vi "Day 10-1.vi"() -> ()   [LabVIEW 2020]
uses:
  Open Symbol.ctl
  <vilib>/regexp/Match Regular Expression.xnode
panel:
  out "Answer":u64
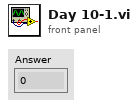
[diagram p1: front panel]
types:
  T1 = typedef "Open Symbol.ctl" = enum16{"(", "[", "{", "<"}
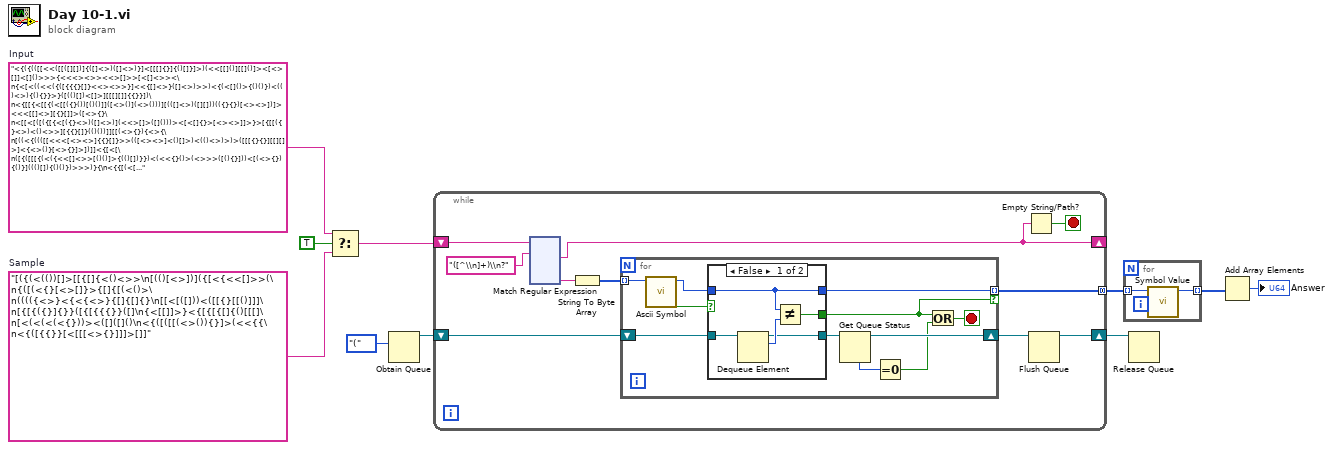
[diagram p0: block diagram]
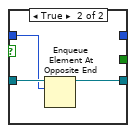
[diagram p2: hidden frame]
diagram:
  w9 = "[({(<(())[]>[[{[]{<()<>>\n[(()[<>])]({[<{<<[]>>(\n{([(<{}[<>[]}>{[]{[(<()>\n(((({<>}<{<{<>}{[]{[]{}\n[[<[([]))<([[{}[[()]]]\n[{[{({}]{}}([{[{{{}}([]\n{<[[]]>}<{[{[{[]{()[[[]\n[<(<(<(<{}))><([]([]()\n<{([([[(<>()){}]>(<<{{\n<{([{{}}[<[[[<>{}]]]>[]]"  # Sample
  w10 = "<{({(([[<<([[([][])]{([]<>)([]<>)}]<[[[]{}]{()[]}]>)(<<[[]()][[]()]><[<>[]]<[]()>>>{<<<><>><<>[]>>[<[]<>><\n{<[<((<<({([{{{}[]}<<><>>}]<<{[]<>}([]<>)>>)<{(<[]()>{()()})<(()<>){(){}}>}([(()[])<[]>][[[][]]{{}}])\n<{[[{<[[{(<[[({}())[()()]]([<>()](<>()))][(([]<>)([][]))(({}{})[<><>])]><<<[[]<>][{}[]]>([<>{}\n<[[<[([({[{<[({}<>)([]<>)](<<>[]>([]()))><[<[]{}>[<><>]]>}>[{[[({}<>)<()<>>][{{}[]}(()())]][[(<>{}){<>{\n[((<{((([[<<<[<><>]{{}[]}>>(([<><>]<()[]>)<(()<>)>)>([[[{}{}][[][]>]<{<>()}[<>{}]>])]]<{[<[\n([{([[[{(<({<<[]<>>[()()]>{(()[])}})<(<<{}()>(<>>>([(){}]))<[(<>{}){()}]((()[]){()()})>>>)}{\n<{{[(<[<<[[{<(()[])>[[{}()]{{}[]}]}[[(<>())[()()]]{<{}{}>}]](<{[<><>]{{}{}}}<({}[])[<><>]>><{[{}<>](<><>)\n{({<[<([[(({({<>()}{{}{}})})<<<((){})[[]()]><{{}()}[[][]]>>{(<{}{}>{{}()})}>)<<{<[{}[]][{}{}]>([[][]]{\n{[(((((<{[({<{()[]}(()())>{<(){}>{{}()}}}(<[<>()]{[]()}>(<()()>{{}<>})))[<[[{}{}](<>()>]({[]<>\n(([((<{<[((<{{<><>}{[]{}}}><<<<>>[{}]>([[]{}]<<>[]>)>)[[{<{}>{()()}}[[{}[]](()()>]](<<<>{}>[[]\n{<([[{<{([[<([[]<>]({}{})){{{}()}({}[])}>](<(<()()><()[]>)<<[]<>>([]{})>>)]){[{<<[()[]]<<>{}>><({\n<{[[([<<<(<{{(()<>)(()())}([{}<>]((){}))}>)>({({{{()<>}({}<>)}<[[]<>]{<>[]}>})(({<(){}>[<>[]]}<([]{})<[]{}>>)\n(<{<{[[({(<[((<>[]){{}})<(<><>)<[]{}>>]((<<>[]><[]()>)<<{}{}>{(){}}>)>(<[[[]<>]]{{<>{}}{[]()}}>(<{\n{(({{[[{<[((<<()<>>[{}{}]>((()<>){[]()})){{(<>{})[<>[]]}<<<><>>>}){{({<>{}}([]()))[{<><>}{[]\n(([<(([({{<{[{()<>}<{}[]>]}{[[()()][()<>]}[{<>{}}({}{})]}>((<<<>{}>[<>()]>{{[]<>}({}{})}){[<{\n[[{{(<<[[[[<<<<>{}>({}())>[([]<>)(()())]>]<<<{<>()}>[<<>[]>[()()]]>[([[]()]<[][]))<[<>{}]{{}<>\n{[{(((([<[{([(()()){()()}][<(){}>[{}<>)])[(<{}<>>{<>()})({{}<>}[()[]])]}(<({[]<>}<()[]>)({[]<>\n<<([(([{<{<<<[{}[]]((){})>((<>[])(()<>))>{{{<>()}{[]}}{([][])}}>[<{{<>[]}<<>>}({[]<>})>]]({({{<><>\n[{((<{<[[<[{[{{}<>}]{[{}][<>[]]}}[<([]())<()[]>>((<>){[]{}})]]<{(<()<>><{}<>]){[[]<>]({}{})}}({<{}[]>{{}\n<[<{(<[[<(((<({}[])><(<><>)(<>())]){{{()()}(<>())}<[{}()]>})[([[<>[]]{{}[]}]{{{}()}<{}[]>})[[(()<>){<>\n[([{{[<([{[([[()<>]])([[<>][()[]]][[<>[]]<<>[]>])]}{([<<{}()>({})>(<[]()>(<><>))]<<{{}<>}{<>}><(<>\n<<[[([([(<(<<[{}[]]<()[]]><{[]{}}[<>()]>>)>[<<({[][]}<<><>>)[<{}{}>{()<>}]><({<>{}}([]))((\n<({<{(<[({([[{()}(<><>)](<[][]>[{}{}])](([[]<>]<<>{}>))){({<<>{}>[[]{}]}<([][])>)<<(<><>)<[]<>>}>}}((([[()<\n{([<(<[(({[({[(){}]<<>{}>}[[{}{}][{}[]]])]{({[()<>]{()[]}}(<[][]>[()[]])){{{[]{}}(<>[])}[<(){}>(\n<[<[<{[{<[{[<<{}<>>(<>)>]{<({}{}){(){}}>((<>{})[{}<>])}}[<[[<><>]{{}<>}]{<()()>}>{<<[]()>(()())>{{{}<\n(({[[<<[({[{{<()()>}}{<[<>()]>}][(<{[][]}>{[{}()]{[]<>}})<{{<>{}}(()[])}{{[]()}<<>[]>}>]})\n<((<([[({(<{[[(){}]<[][]>]}>({<[()<>](()[])>(([]<>)([]<>))}<{[[]<>]{(){}}}(<()<>>([][]])>))}<{[<[({}\n{({{{[[{{[{(<<(){}>[{}{}]>((()<>)[<>{}]))[<<{}[]><[]>>[{{}{}}(<>[])]]}[(<<(){}>({}{}))((<>{})([]<>)))\n[[(({[{(<({[{<[]()>{()[]}}<(<>())<()()>>]<(({}[]){{}<>])((()<>){{}[]})>}([[({}{})[<>()]][{<><>}]]{([[\n[[{<[([<[((<([[]{}][{}<>])([{}<>])>[([()<>]{{}{}}){{[]()}}])<({{[]()}[[]()]))>)([<<<<>{}><{}()>><(<>\n<<({{{<{[<{<{<[]<>>[[]{}]}[<[]()>{[]{}}]>[[[(){}][<><>]]{(<>[]}({}{})}]}><[[({{}[]}{[]()}){(<>())[()<\n{{(({[[[{<[<(([]())([]{}))([{}{}](()[])}>]>}([<{[[[]()][(){}]]<{<>[]}>}({<()<>><[]<>>})>((([()\n(<(({{(([(({{<{}[]>({}())}([<>[]][{}()])}((<[][]>{()<>}){[[]<>]<{}{}>}))<({{[]<>}([][])}{<[]{}>{<>[]}})\n((([<([([{{{<<<>{}><{}[]>>[[<>[]][{}[]]]}}(([<<>{}>[()[]]][{{}{}}])(<[()()][<><>]>{{<>[]}})}}]<{[[<\n{{(<[<[<[<<[[(<>[])]({<><>}[()()])]>>]>[{{[[{(<>[])([][])}{[[][]]([]())}]>[[[<{}{}>({}())]<{<>\n<[{[[([[{[(<[<{}{}>{(){}}][{[]<>}<()[]]]>(([()<>][[][]]){[<>{}](()[])}))[[<<{}>[<>{}]>[({}{})({}{})]]<([[]{}\n({<<<{<({{{{{[()()]({}())}[[[]{}][<><>])}({<()()><[]()>}({<>()}))}{(((<>()){()()}){<(){}><()[]>})(([{}()]\n([<({[{({(<<{[{}()]}{{{}[]}((){})}>>)<<{[((){})[()]]}<<{[]<>}<<>()>>([<>()][[]<>])>>{<<[<>[]]<[]<>>)<{<\n(<[<<(<[[[[{{({}<>)[{}{}]}<[[]{}]([]<>)>}][<[<<>{}>{[]}][[[]{}](<>())]><<[<>()][(){}]><{[]\n(({[[(([<(([{({}[])[<>{}]}{(<>[])({}{})})<<<{}[]>({}())>[({}<>)<{}()>]>)[<<[[][]]((){})><{{}(\n{[((<([<[{[{<[<><>][()()]><{<>{}}>}[{<[][]>[()<>]}<(<>())<()<>>>]]<<<(<>())<()[]>>>[{{{}[]}}[[{}()]((){\n{{<{({{({[<((({}{}){<>[]}){<{}()>{<>[]}})>(<{<<>{}><[]<>>}>[[{[]<>>{<><>}]{((){})<(){}>}])]}(<{[{{<><>}{[\n(({<[[{[(<(((({}{}){()<>}))<{{[]{}}{{}{}}}<[{}<>][(){}]>>)>[{{(<<><>>([]{}))[((){})<{}[]>]}}(([[<>()]{<>()}]\n[<([[[<[<{<{<{[]{}}{[]{}}>[([]())<<>[]>]}({{[]{}}<[]()>}<({}())(<>{})>)>}[({[[{}[]][{}<>]]})]>]><[\n<{[<<[[<{[[{<<{}[]>[<><>]>}({[[]{}]<{}()>}((()[])))]{[<{()}[[]{}]>]{(({}[])<{}()>)<(<>())[()<>]\n[[([[{[[(([{[[<>()]{<>()}]({(){}}({}{}))}[<[<><>]([]())>(<[]()><{}[]>)]]{(<<<><>>[[]{}]>(<[][]>((){}))\n{(<<[[{[{{(<<<{}[]>(<>[])>({[]{}}([]{}))>[{<<>()>[[]<>]]([{}[]])])}[[{(<<><>>[()()])<<<><>>>}([<<>\n([((<(<[(<{((<{}{}>{<><>})){{(()[])[{}[]]}}}{[[[(){}][<><>]]]({<()<>>{{}[]}}<[()()]{()[]}>)}>[<{(<{}\n[(<[([[({({<[{<>()}([]<>)][(<><>)<()[]>]>})[{([(())({}[])][{[]<>}<()<>>])}({<[{}{}](()())><({}())[<>[]\n([(<<[<{<{((<(<>[])({}<>)>{{()()}<<>{}>}))<{[[()[]][()[]]][({}[])<{}()>]}{<({})><{[][]}{{}<>}>}>}<<<({(){}}\n[(<{(([({<{{(<[]<>>({}()))}}[<[[{}[]][[]]]>[({[]<>}(<>{}))]]>})]<([(<([[()()][[][]]]<((){}\n((({([(<<{{<<({}())(())>([<>()]<()()>)>}}<[(<{{}[]}<()<>>><({}{}){(){}}>)][(({()<>}([]()))([()]))({{{}()}\n{<(({[<([{[({([][])[[]{}]}<({}<>)<<>()>>)<<{<>()}{[]<>}>{{{}}{[]()}}>]}])<<{<(([[]{}]<<>[]>)){<<[]<>>><<()[\n[{<(<<<((<<<{[()<>]{[]<>}}>[[<{}{}>[()[]]]<(<><>)[()[]]>]>{[[[[]()][<>[]]]]({(<>}{[]{}}})}>){({\n<<[((<<[{{[(<[<>()]><{{}[]}{<>{}}>){[(()[])([]())][[(){}][{}[]]]}]([<[[][]]{(){}}><<{}{}>{<>{}}>][[\n{<<{<<{<({[[([<>{}])[{[]<>}{{}[]}]][[<()<>>[<>{}]]]]<([{[]()}({}{})]({[]()}{<>()})){[({}<>)[[]{}\n{<<[{((([<([[<[]()><<><>>][{()<>}<[][]>]]{<[{}[]][()[]]>[{<>{}>{[]}]}){[([[]{}]<()[]>)[[<>()][{}[]]\n({{{{<([[((({{{}{}}<()[]>}{<()<>>{{}<>}})(<({}{})>({<>{}}[[]()]))){(<<<><>><()[]>>[{()()}{[]<>}\n({<{[[{({{[<[{[][]}<[][]>]{(<><>)}>([[<>{}][<>{}]]({[]{}}<<>[]>))]}{[({[[]]{()[]}}{(<>{})[()()]})(<{(\n[{<<<[(<(<{((([]{}))[{<>()}[()[]]]){{<{}{}>}[<[]<>>{<>{}}]}}<(<[<>[]][()()]>)<([{}()]{{}[]})\n{{(([[([((<([[<><>]])>({[{()<>}<[]{}>]}<{[()()]<{}>}(<{}<>>({}{}))>))[{{([()()]<{}<>>){(<>{})(\n([(<{[[{<{{<{([]())(<>[])}{{[]<>}{()<>}}>{{{()}}[<[]{}><{}<>>]}}<{[{()()}]{{<>[]}[<><>]}}<<{<>(\n([[{[{[{<<(<{<{}{}>{[]}}{[{}{}]{()[]}}>[{({}[])}<[()[]]>])>>[(<<({<>{}}{[]{}})>>(<[([]()){()<>}]((()())([]\n(({<({<([(({<<<>()>([]())>{<()[]>{[]<>}}}(<{{}<>}[()()]>({{}<>}[{}()]))))]){{<[{[(<>[]){()\n([[(<{[[{<[<(<[]()>[{}[]]){[<><>]{<>[]}}>{{([]()){[]{}}}<((){})([]<>)>}]<<<{{}[]}[()]>(<{}><[][]>)>>>}\n{{(<[{[([<<<[<{}<>>(<>{})]<({}[])[<>[]]>>({<{}{}><[]{}>}<<[]><(){}>>)>>(((({()()}[[]{}]))<[{[]<>)<[]()>]\n(({{<<[{([[({[[]{}]{()<>}}[(<><>)[()()]])[<[<>[]]><([]{})[[][]]>]](<((<><>)<<>()>)[([][])((){})]>[(\n((<<([[<{[{({<(){}><[][]>}{(()[])({}[])})({[{}()]({}{})}(<(){}>(<><>)))}{{[{()<>}<{}{}>][{[]{}}(()\n<{(((([<[((({{{}<>}[[]<>]}<[{}<>]>)[<({}{})>{{[]()}<{}()>}])<([<<>>(<><>)]((()())(<>{})))>){(({(\n<{{<<{{{[({{[<()[]>(()[])]}<<[[]<>][[]]>>}[<[({})<<>[]>][[[]]([][])]>])]}}(<({[[<[(){}]>{<[]{}>}]{(({\n[([[(({([{{({{()}[{}<>]}{({}<>){{}()}}]}}{[<<({}())<(){}>>[{()[]}([]{})]>]{<<{{}()}(<>[])>{[(\n[{[{[([<<((<<{()<>}<<>()>>[{[]{}}{{}[]}]>[[{[][]}{{}}]])(([((){})(()())]{[(){}]{()}})))}{(<<<<<><>>({}[]\n<[{({[({[({{(<[]()>{{}<>}){{{}<>}[(){}]}}(([{}()]<[][]>)[[<>]({}{})])}<<[(<>)({})]<<()[]><\n[((([<(({<<({{{}()}({}<>)}({()[]}[{}{}]))>{[{(<>[])}{(<>[])<{}[]>}]{<[<><>][()[]]>}}>({<{<<>()><<><>>}([{}[]]\n{({((<<([((<[[()[]]{[][]}]<{(){}}{<>{}}>>({[(){}][<>]})))(<(({<>[]}<(){}>)(<()[]><{}()>))>)]){\n<{<[<(<{<[({{{{}<>}<<>{}>}{[[]()][{}{}]}}[({<><>}{<>{}})[[{}()]{[]()}]])({{<[])(<>[])}})](<<[[<><>]](<{}{}>\n[([[[{[((<<(<<()()>>)><<{([]()){<>{}}}<{[]{}}<()()>>>[(<<><>>[()[]]){((){})([]{})}]>>({[<[<><>]{<><\n<{{({{{[<{[{{{()<>}[<><>]}[(()[]){[]{}}]}(<{{}[]}[<>[]]><{{}{}}<{}[]>>)]{(({(){}}<<>{}>)[<<><>>[{}\n[[([[{[({[{[({{}[]}{()[]})[<()()>{{}{}}]][(([]<>)<[][]>)[<{}{}><{}()>]]}][<([([][]){()()}][[{}{}]{()<\n{(<<(((<((((<{()<>}<<>[]>)[<[][]>[{}()]]){[[[]<>]<(){}>][<()<>>{{}<>}]})))<[{{[{{}{}}<[]<>>]}}(\n{[(<{[<{{({[{[<><>](<>{})}{({}[])(<>{})}]}({<({}[])<[]<>>>(({}[]))}[<<()><<>>}[{()[]}{[][]}]])){[({<<>()>(\n<([{[(<(<<([((()())<{}{}>)]<{(<>())(<>()]}{[()<>](<>())}>)<[[<[][]>]{{()}<<><>>}](({()()}[[\n<[<[<{{{[{((<(()()){{}<>)><[[]()](()<>)>))({[[<>{}]{{}()}]({()<>}(()[]))})}]}([{((({{}()}[()<\n[{([({[<(<{[{[<>[]][<>()]}([[]{}](()()))){{[()()]<(){}>}({()[]}<[]()>)}}<{[(<>[]){()<>}][[()<>]{()[]}]}{<(<>\n{((<(<({{([{[([]<>){[]<>}](<[]<>>[[]<>])}{{<[][]><()[]>}({()<>}<<>{}>)}]<[<[<>()]([]{})><{{}<>}<{}<>>>][(\n{<<([<(<{[[{{{<>[]}[[]<>]}{[{}[]]]}{<[(){}]>{[{}()]{[]<>}}}](<{[[]<>]{<>[]}}<<()<>>[[]()]>>)]<[{{<{}>[{}]}<(\n[[{{{<{[{({<<<[]{}>[()<>]><[[]<>]([]<>)>><{<<>()>[<>{}]}>}((<[{}{}]{[]}]{<[]<>>{<>{}}})[([<>(\n[[{<<{{[(([[[{()[]}][[()[]]<[]>]]({{{}}})][({([][])[{}{}]}<[(){}]<()[]>>){<{[]{}}[(){}]><{{}{}}<<>()>]}]))<<\n[(({[<<{<({<([<><>])[{<>()>{{}[]}]>((<()<>><{}<>>)[{[][]}([]{})])})<{{([[]<>]<{}<>>)([()[]]{()()}\n[([(({(<[<[<((<>{})[[]<>]){[<><>]({}[]>}>]>]>)}[(({(<<[{(){}}[()[]]]>[<(<>{}){{}{}}>[[()<>][()]]]>)\n{<{{<({<{((<{({})<<>{}>}((()){()<>})>))}((<{((()[]){{}[]})[<<>>[[]<>]]}(([<>](()<>)))><{{{<>()}((){}}}((\n<[<{<((({{[<{{[][]}}<([]<>)(<>{})>>]}[(([{()()}{<>()}])[<[()[]][()[]]>]){<<[<>()](<>{})>{{(){}}(<>\n(([{([{[<(<(((()<>))[(())(<>{})])([[{}<>]{{}[]}][{<><>}[{}{}]])>[(([()[]]<[][]>)[{{}[]}(()[])])(([{}{}]\n{<(<<{<[{<{<<<<>[]>[[]<>]){[[]()][<><>]}>({(<><>)(()<>)})}>[<([{{}{}}<[]<>>])({{[]<>}({}[])})>]}{<<[(\n<{([({{{<{[{(([]())<<><>>)<[()()]((){})>}]}(<{(<(){}>(<>()))}([[()[]][(){}]](<<>{}>[{}()])}>)>([{<(\n((([{<<[{{[(<<[]<>>(<>())>{({}{})<{}[]>})[[<()()>[<>[]]][<{}[]>(()())]]]}}]>>)]{{{{[[{[[[([]<>){\n({(<{{({[[{<<(()[])[()]>[{<><>}{<>[]}]>{<{<><>}{()[]}>{[{}()]{[][]}}}}{<<{[]<>}(<><>)>{{[]{}}[\n(<[{{(([<{{(<[<>()]((){})>{<{}[]>({}())})}}>][<[{{([{}[]])<([]<>)<<>{}>>}}{<({[][]}(()()))(<<>()>{\n(<<{{{((<{({<<{}()><{}{}>><<()[]>[<>[]]>>(<[(){}]([]<>)>[({}<>)]))(({{[]<>}<()<>>}[<()[]>(()[])]){<[\n<[(((<({([({{[[]()]{[]()}}([{}()]<[]<>>)}[[<()[]>{{}{}}]([<>]<<>()>)]){[((()<>){<>[]}){[{}[]){[\n(({[[({{{[{{({(){}}{{}[]})<({}[])([]<>)>}[[(<>{})]<([]()){{}()}>]}[{<{[]<>}<()()>>([{}<>]<{\n<[({{[<[{({[({[]<>}{{}[]})[{[][]}{[][]}]][[<{}[]>{[]()}]([()[]]({}<>))]}{<{[{}<>]<[]()>}<<[]()>[<>{}]>><((\n[{[{<{{[<<[[<<{}<>>>][{{{}[]}({}())}]]([{<<><>>({}{})}{{[]<>}}]{{{[]()}([]<>)}})><({{<[][]>}}){<{{()><()>}>[<\n{{({([<({(<[({{}{}}<[]{}>)]>[(((<>()){<>()]))[<({}[])(<>{})>{<<><>>{[]()}}]]){{[<(()[])<()<>>>(<()<>>)]([<{}\n[({[<(<<[{<({<{}()>{{}()}})({({})<()()>}[{[]<>}[{}{}]})><[(({}{}))(((){})[[][]])]>}<{([<[]<>>]<[{}[]]((\n[<{{{<<(<[[{<([][]){<>}>}{<[[]]{[]{}}><{<>{}}>}]<<{([]())[<>[]]}><(([]{}){[]<>})[(<>())({}<>}]>>]("  # Input
  n1 = Select(t=w10, s=TRUE, f=w9) -> (s? t:f=w7:string)
  n2 = Obtain Queue(element data type=Open_Symbol."(" ("Open Symbol")) -> (queue out=w5:refnum<queue>)  [unwired: 4 in, 2 out]
  n3 = while {
    shift-right: [w18] -> _
    shift-left: w7 -> [w20]
    shift-right: [w12] -> w4
    shift-left: w5 -> [w14]
    tunnel: [w11] -> w3 mode=concatenating
    stop <- w17 stop-if-true
    n4 = xnode "Match Regular Expression"("input string"=w20, "regular expression"="([^\\n]+)\\n?") -> ("after match"=w18:string, "submatch 1"=w16:string)  [unwired: 4 in, 4 out]
    n5 = String To Byte Array(string=w16) -> (unsigned byte array=w15:u8[])
    n6 = for {
      tunnel: w15 -> [w31] mode=indexing
      shift-right: [w25] -> w13
      shift-left: w14 -> [w28]
      tunnel: [w26] -> w11 mode=indexing if=w23
      stop <- w21 stop-if-true
      n7 = call "Ascii Symbol.vi"("Character"=w31) -> ("Symbol"=w29:T1, "Open"=w30:bool)  [unwired: 9 in]
      n8 = case shown="False" w30 {
        tunnel: w29 -> [w34 w38]
        tunnel: w28 -> [w36 w39]
        tunnel: [w32 w37] -> w27
        tunnel: [w34 _] -> w26
        tunnel: [w33 _] -> w23
        frame False {
          n9 = Dequeue Element(queue=w36) -> (queue out=w32:refnum<queue>, element=w35:T1)  [unwired: 2 in, 2 out]
          n10 = Not Equal?(x=w34, y=w35) -> (x != y?=w33:bool)
        }
        frame True {
          n11 = Enqueue Element At Opposite End(queue=w39, element=w38) -> (queue out=w37:refnum<queue>)  [unwired: 2 in, 2 out]
        }
      }
      n12 = Get Queue Status(queue=w27) -> (queue out=w25:refnum<queue>, # elements in queue=w24:i32)  [unwired: 2 in, 6 out]
      n13 = Equal To 0?(x=w24) -> (x = 0?=w22:bool)
      n14 = Or(x=w23, y=w22) -> (x .or. y?=w21:bool)
    }
    n15 = Empty String/Path?(string/path=w18) -> (empty?=w17:bool)
    n16 = Flush Queue(queue=w13) -> (queue out=w12:refnum<queue>)  [unwired: 1 in, 2 out]
  }
  n17 = for {
    tunnel: w3 -> [w157] mode=indexing
    tunnel: [w156] -> w2 mode=indexing
    n18 = call "Symbol Value.vi"("Open Symbol"=w157) -> ("Corrupt Value"=w156:u64)  [unwired: 9 in, 1 out]
  }
  n19 = Release Queue(queue=w4) -> ()  [unwired: 2 in, 3 out]
  n20 = Add Array Elements(numeric array=w2) -> (sum=→"Answer":u64)
